vi "InvertMatrix.vi"(3 "A":T1={"nx"=1.0, "ny"=0.0, "nz"=0.0, "nw"=0.0, "ox"=0.0, "oy"=1.0, "oz"=0.0, "ow"=0.0, "ax"=0.0, "ay"=0.0, "az"=1.0, "aw"=0.0, "Px"=5.0, "Py"=2.0, "Pz"=3.0, "Pw"=1.0} {"Pw" format="%.2f"; "Pz" format="%.2f"; "Py" format="%.2f"; "Px" format="%.2f"; "aw" format="%.2f"; "az" format="%.2f"; "ay" format="%.2f"; "ax" format="%.2f"; "ow" format="%.2f"; "nw" format="%.2f"; "oz" format="%.2f"; "oy" format="%.2f"; "ox" format="%.2f"; "nz" format="%.2f"; "ny" format="%.2f"; "nx" format="%.2f"}) -> (0 "error":i32, 1 "Inverse of A":T1={"nx"=1.0, "ny"=0.0, "nz"=0.0, "nw"=0.0, "ox"=0.0, "oy"=1.0, "oz"=0.0, "ow"=0.0, "ax"=0.0, "ay"=0.0, "az"=1.0, "aw"=0.0, "Px"=0.0, "Py"=0.0, "Pz"=0.0, "Pw"=1.0} {"Pw" format="%.2f"; "Pz" format="%.2f"; "Py" format="%.2f"; "Px" format="%.2f"; "aw" format="%.2f"; "az" format="%.2f"; "ay" format="%.2f"; "ax" format="%.2f"; "ow" format="%.2f"; "nw" format="%.2f"; "oz" format="%.2f"; "oy" format="%.2f"; "ox" format="%.2f"; "nz" format="%.2f"; "ny" format="%.2f"; "nx" format="%.2f"})   [LabVIEW 2010]
uses:
  <vilib>/Analysis/NI_AALBase.lvlib
  <vilib>/Analysis/baseanly.llb/Real Inverse Matrix.vi
  ReferenceFrame.ctl
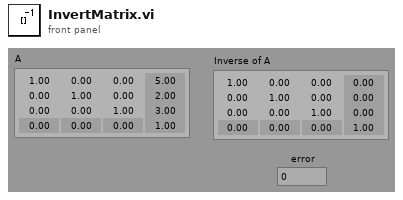
[diagram p1: front panel]
types:
  T1 = typedef "ReferenceFrame.ctl" = cluster{"nx":dbl, "ny":dbl, "nz":dbl, "nw":dbl, "ox":dbl, "oy":dbl, "oz":dbl, "ow":dbl, "ax":dbl, "ay":dbl, "az":dbl, "aw":dbl, "Px":dbl, "Py":dbl, "Pz":dbl, "Pw":dbl}
  T2 = typedef "NI_Matrix.lvlib/RealMatrix.ctl" = dbl[][]
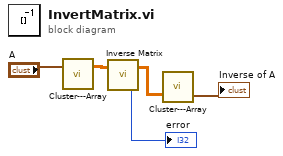
[diagram p0: block diagram]
diagram:
  n1 = call "Cluster---Array.vi"("A"="A") -> ("Array (A)"=w3:dbl[][])  [unwired: 1 in, 1 out]
  n2 = call-poly <vilib>:"Inverse Matrix.vi"("Input Matrix"=w3) -> ("error"=→"error":i32, "Inverse Matrix"=w1:T2)  [unwired: 1 in]
  n3 = call "Cluster---Array.vi"("Array (A) in"=w1) -> ("A"=→"Inverse of A":T1)  [unwired: 1 in, 1 out]
